vi "Merge_Localization_Settings_in_Cluster-1.vi"(4 "[IN] Binarization Settings":cluster{"MinBin2":sgl, "MaxBin2":sgl}[](array[cluster]), 5 "[IN] AVI Refnum":T1, 6 "[IN] Image Filtering Settings":T5, 7 "[IN] Image Type":T2 items=["Grayscale (U8)", "Grayscale (I16)", "Grayscale (SGL)", "Complex (CSG)", "RGB (U32)", "HSL (U32)", "RGB (U64)", "Grayscale (U16)"], 9 "[IN] Keep Nega-\ntive Values?":bool, 10 "[IN] # Channel":u8=1, 11 "[IN] Particle Filter Setups":T6 {"Type of particle filter"."Measurement Parameter" items=["Center of Mass X", "Center of Mass Y", "First Pixel X", "First Pixel Y", "Bounding Rect Left", "Bounding Rect Top", "Bounding Rect Right", "Bounding Rect Bottom", "Max Feret Diameter Start X", "Max Feret Diameter Start Y", "Max Feret Diameter End X", "Max Feret Diameter End Y", "Max Horiz. Segment Length Left", "Max Horiz. Segment Length Right", "Max Horiz. Segment Length Row", "-", "Bounding Rect Width", "Bounding Rect Height", "Bounding Rect Diagonal", "Perimeter", "Convex Hull Perimeter", "Holes' Perimeter", "Max Feret Diameter", "Equivalent Ellipse Major Axis", "Equivalent Ellipse Minor Axis", "Equivalent Ellipse Minor Axis (Feret)", "Equivalent Rect Long Side", "Equivalent Rect Short Side", "Equivalent Rect Diagonal", "Equivalent Rect Short Side (Feret)", "Average Horiz. Segment Length", "Average Vert. Segment Length", "Hydraulic Radius", "Waddel Disk Diameter", "-", "Area", "Holes' Area", "Particle & Holes' Area", "Convex Hull Area", "Image Area", "-", "Number of Holes", "Number of Horiz. Segments", "Number of Vert. Segments", "-", "Orientation", "Max Feret Diameter Orientation", "-", "% Area/Image Area", "% Area/(Particle & Holes' Area)", "Ratio of Equivalent Ellipse Axes", "Ratio of Equivalent Rect Sides", "-", "Elongation Factor", "Compactness Factor", "Heywood Circularity Factor", "Type Factor", "-", "Sum X", "Sum Y", "Sum XX", "Sum XY", "Sum YY", "Sum XXX", "Sum XXY", "Sum XYY", "Sum YYY", "-", "Moment of Inertia XX", "Moment of Inertia XY", "Moment of Inertia YY", "Moment of Inertia XXX", "Moment of Inertia XXY", "Moment of Inertia XYY", "Moment of Inertia YYY", "Norm. Moment of Inertia XX", "Norm. Moment of Inertia XY", "Norm. Moment of Inertia YY", "Norm. Moment of Inertia XXX", "Norm. Moment of Inertia XXY", "Norm. Moment of Inertia XYY", "Norm. Moment of Inertia YYY", "Hu Moment 1", "Hu Moment 2", "Hu Moment 3", "Hu Moment 4", "Hu Moment 5", "Hu Moment 6", "Hu Moment 7"]}) -> (2 "[OUT] Localization Settings":T4 {"[IN] Image Type" items=["Grayscale (U8)", "Grayscale (I16)", "Grayscale (SGL)", "Complex (CSG)", "RGB (U32)", "HSL (U32)", "RGB (U64)", "Grayscale (U16)"]; "[IN] Particle Filter Setups"."Type of particle filter"."Measurement Parameter" items=["Center of Mass X", "Center of Mass Y", "First Pixel X", "First Pixel Y", "Bounding Rect Left", "Bounding Rect Top", "Bounding Rect Right", "Bounding Rect Bottom", "Max Feret Diameter Start X", "Max Feret Diameter Start Y", "Max Feret Diameter End X", "Max Feret Diameter End Y", "Max Horiz. Segment Length Left", "Max Horiz. Segment Length Right", "Max Horiz. Segment Length Row", "-", "Bounding Rect Width", "Bounding Rect Height", "Bounding Rect Diagonal", "Perimeter", "Convex Hull Perimeter", "Holes' Perimeter", "Max Feret Diameter", "Equivalent Ellipse Major Axis", "Equivalent Ellipse Minor Axis", "Equivalent Ellipse Minor Axis (Feret)", "Equivalent Rect Long Side", "Equivalent Rect Short Side", "Equivalent Rect Diagonal", "Equivalent Rect Short Side (Feret)", "Average Horiz. Segment Length", "Average Vert. Segment Length", "Hydraulic Radius", "Waddel Disk Diameter", "-", "Area", "Holes' Area", "Particle & Holes' Area", "Convex Hull Area", "Image Area", "-", "Number of Holes", "Number of Horiz. Segments", "Number of Vert. Segments", "-", "Orientation", "Max Feret Diameter Orientation", "-", "% Area/Image Area", "% Area/(Particle & Holes' Area)", "Ratio of Equivalent Ellipse Axes", "Ratio of Equivalent Rect Sides", "-", "Elongation Factor", "Compactness Factor", "Heywood Circularity Factor", "Type Factor", "-", "Sum X", "Sum Y", "Sum XX", "Sum XY", "Sum YY", "Sum XXX", "Sum XXY", "Sum XYY", "Sum YYY", "-", "Moment of Inertia XX", "Moment of Inertia XY", "Moment of Inertia YY", "Moment of Inertia XXX", "Moment of Inertia XXY", "Moment of Inertia XYY", "Moment of Inertia YYY", "Norm. Moment of Inertia XX", "Norm. Moment of Inertia XY", "Norm. Moment of Inertia YY", "Norm. Moment of Inertia XXX", "Norm. Moment of Inertia XXY", "Norm. Moment of Inertia XYY", "Norm. Moment of Inertia YYY", "Hu Moment 1", "Hu Moment 2", "Hu Moment 3", "Hu Moment 4", "Hu Moment 5", "Hu Moment 6", "Hu Moment 7"]})   [LabVIEW 2017]
doc: "The subVI provides additional merging of settings"
uses:
  <vilib>/vision/Avi.llb/IMAQ AVI2 Refnum.ctl
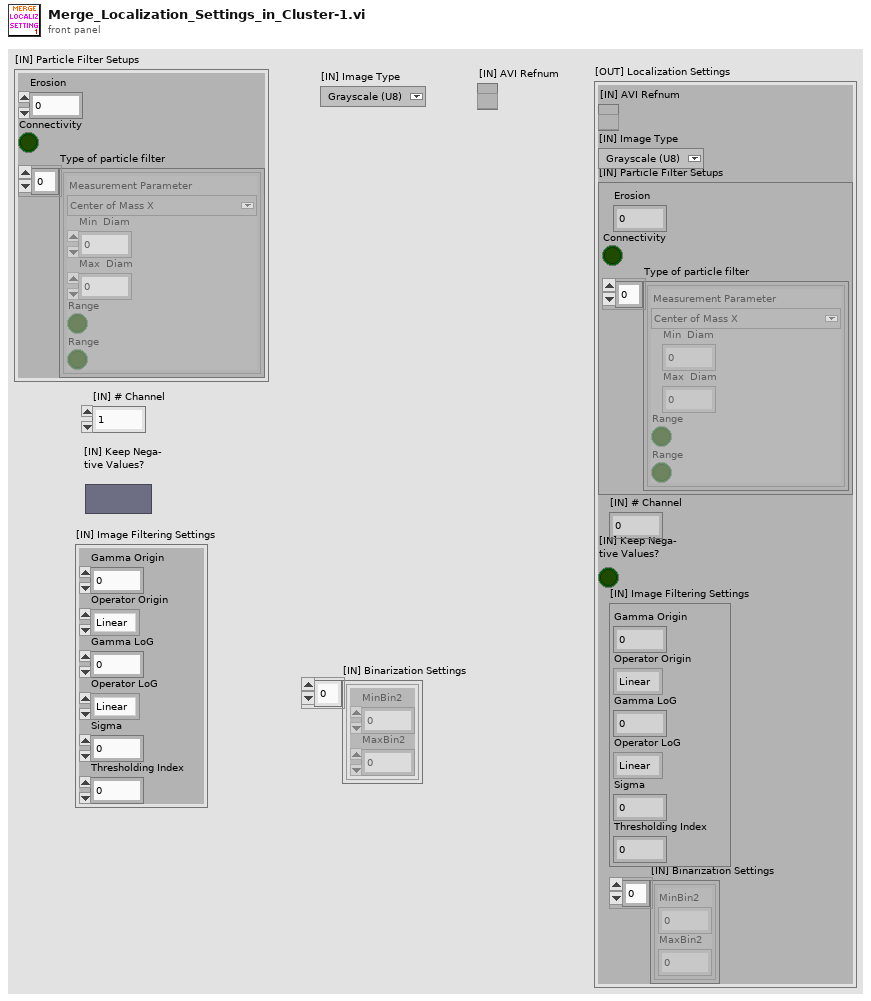
[diagram p1: front panel]
types:
  T1 = typedef "IMAQ AVI2 Refnum.ctl" = refnum<k20>
  T2 = typedef "Image Type" = u32
  T3 = typedef "Particle Parameters" = i32
  T4 = cluster{"[IN] AVI Refnum":T1, "[IN] Image Type":T2, "[IN] Particle Filter Setups":cluster{"Erosion":i32, "Connectivity ":bool, "Type of particle filter":cluster{"Measurement Parameter":T3, "Min  Diam":dbl, "Max  Diam":dbl, "Range":bool, "Range":bool}[]}, "[IN] # Channel":u8, "[IN] Keep Nega-\ntive Values?":bool, "[IN] Image Filtering Settings":cluster{"Gamma Origin":sgl, "Operator Origin":enum32{"Linear", "Log", "Exp", "Square", "Square root", "Power X", "Power 1/X"}, "Gamma LoG":sgl, "Operator LoG":enum32{"Linear", "Log", "Exp", "Square", "Square root", "Power X", "Power 1/X"}, "Sigma":dbl, "Thresholding Index":i8}, "[IN] Binarization Settings":cluster{"MinBin2":sgl, "MaxBin2":sgl}[]}
  T5 = cluster{"Gamma Origin":sgl, "Operator Origin":enum32{"Linear", "Log", "Exp", "Square", "Square root", "Power X", "Power 1/X"}, "Gamma LoG":sgl, "Operator LoG":enum32{"Linear", "Log", "Exp", "Square", "Square root", "Power X", "Power 1/X"}, "Sigma":dbl, "Thresholding Index":i8}
  T6 = cluster{"Erosion":i32, "Connectivity ":bool, "Type of particle filter":cluster{"Measurement Parameter":T3, "Min  Diam":dbl, "Max  Diam":dbl, "Range":bool, "Range":bool}[]}
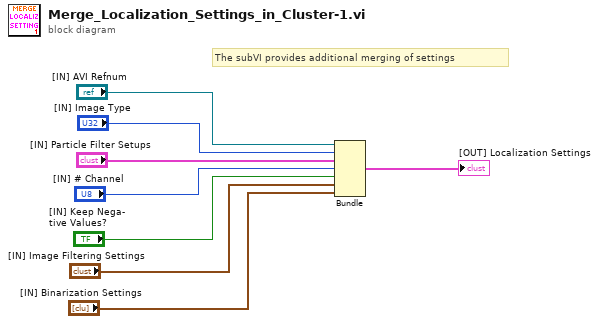
[diagram p0: block diagram]
diagram:
  # "The subVI provides additional merging of settings"
  n1 = Bundle("[IN] AVI Refnum"="[IN] AVI Refnum", "[IN] Image Type"="[IN] Image Type", "[IN] Particle Filter Setups"="[IN] Particle Filter Setups", "[IN] # Channel"="[IN] # Channel", "[IN] Keep Nega-\ntive Values?"="[IN] Keep Nega-\ntive Values?", "[IN] Image Filtering Settings"="[IN] Image Filtering Settings", "[IN] Binarization Settings"="[IN] Binarization Settings") -> (→"[OUT] Localization Settings":T4)  [unwired: 1 in]
